vi "Check Variant Type.vi"(8 "error in (no error)":errorcluster, 10 "Variant In":variant, 11 "Field in":refnum<class "Field.lvclass">) -> (0 "error out":errorcluster, 2 "Variant Out":variant, 3 "Field out":refnum<class "Field.lvclass">)   [LabVIEW 2020]
uses:
  Field.lvclass
panel:
  # "For override: Check that variant type is compatible with field control object"
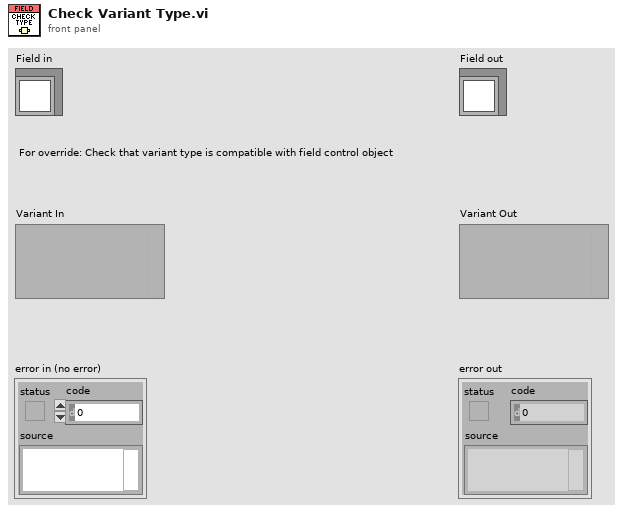
[diagram p1: front panel]
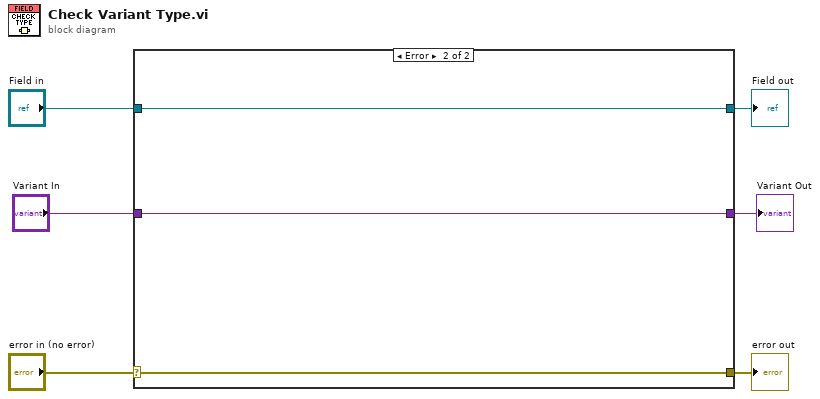
[diagram p0: block diagram]
diagram:
  n1 = case shown="Error" "error in (no error)" {
    selector: "error in (no error)" -> [w8 w12]
    tunnel: [w8 w12] -> w5
    tunnel: [w9 w11] -> w3
    tunnel: "Field in" -> [w9 w11]
    tunnel: "Variant In" -> [w7 w10]
    tunnel: [w7 w10] -> w1
    frame No Error {
      # "Wire the error cluster across even in the \"No Error\"\ncase so that warnings get propagated."
    }
    frame Error {
    }
  }
  "error out" <- w5
  "Field out" <- w3
  "Variant Out" <- w1
